vi "Voltage Read Single.vi"(8 "error in":errorcluster, 9 "Channel Index":i32=1, 11 "Device in":refnum<class "Device.lvclass">) -> (0 "error out":errorcluster, 1 "Changed or First Call?":bool, 2 "Voltage.chX.SP":dbl, 3 "Device out":refnum<class "Device.lvclass">)   [LabVIEW 2023, in "Device.lvclass"]
uses:
  Device.lvclass
  Device.lvclass/Device.ctl
  Low Level Capabilities/Voltage/Voltage Setpoint/Voltage Setpoint.lvclass
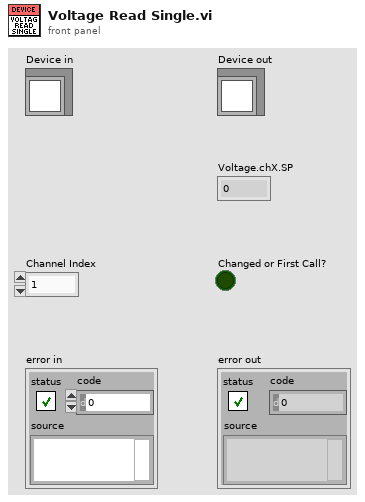
[diagram p1: front panel]
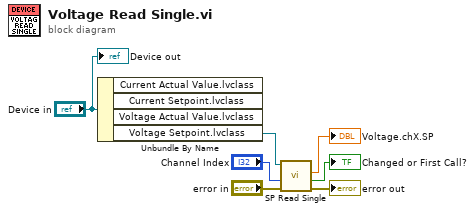
[diagram p0: block diagram]
diagram:
  n1 = Unbundle By Name("Device in") -> ("Voltage Setpoint.lvclass"=w3:refnum<class "Voltage Setpoint.lvclass">)  [unwired: 3 out]
  n2 = call-dynamic "SP Read Single.vi"("error in"="error in", "Channel Index"="Channel Index", "Voltage Setpoint in"=w3) -> ("error out"=→"error out":errorcluster, "Changed or First Call?"=→"Changed or First Call?":bool, "Voltage SP"=→"Voltage.chX.SP":dbl)  [unwired: 5 in, 1 out]
  "Device out" <- "Device in"
